vi "Create All Message Queues.vi"(8 "error in (no error)":errorcluster) -> (0 "error out":errorcluster, 3 "Message Queues out":T1)   [LabVIEW 2015, in "Message Queue.lvlib"]
doc: "This VI creates and initializes all the message queues for your application. If your application requires more than one message queue, right-click the \"Message Queues\" constant above and select Open Type Def. Add the new Message Queue(s) to the type definition, then initialize them in this VI."
uses:
  Message Queue.lvlib
  Message Cluster.ctl
  All Message Queues.ctl
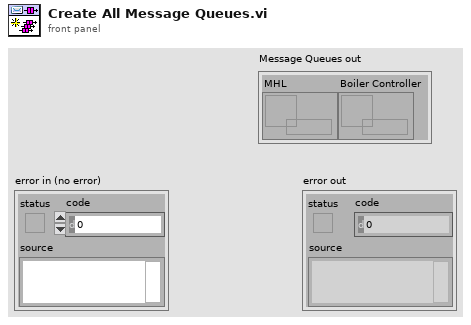
[diagram p1: front panel]
types:
  T1 = typedef "Message Queue.lvlib/All Message Queues.ctl" = cluster{"MHL":refnum<queue>, "Boiler Controller":refnum<queue>}
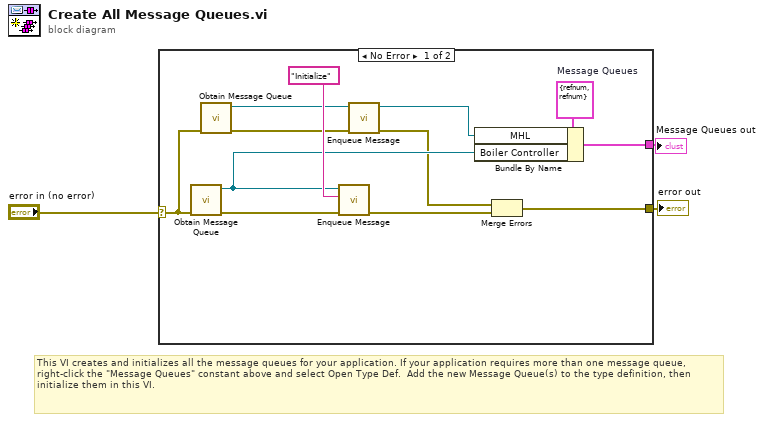
[diagram p0: block diagram]
diagram:
  # "This VI creates and initializes all the message queues for your application. If your application requires more than one message queue, right-click the \"Message Queues\" constant above and select Open Type Def.  Add the new Message Queue(s) to the type definition, then initialize them in this VI."
  n1 = case shown="No Error" "error in (no error)" {
    selector: "error in (no error)" -> [w6 w16]
    tunnel: [w9 w16] -> w3
    tunnel: [w11 _] -> w2
    frame No Error {
      w14 = T1 {"MHL"=refnum, "Boiler Controller"=refnum}  # Message Queues
      n2 = call "Obtain Message Queue.vi"("error in (no error)"=w6) -> ("error out"=w13:errorcluster, "Message Queue"=w10:refnum<queue>)  [unwired: 9 in]
      n3 = call "Obtain Message Queue.vi"("error in (no error)"=w6) -> ("error out"=w7:errorcluster, "Message Queue"=w5:refnum<queue>)  [unwired: 9 in]
      n4 = call "Enqueue Message.vi"("error in (no error)"=w13, "Message"="Initialize", "Message Queue"=w10) -> ("error out"=w15:errorcluster)  [unwired: 7 in, 1 out]
      n5 = call "Enqueue Message.vi"("error in (no error)"=w7, "Message Queue"=w5) -> ("error out"=w8:errorcluster, "dup Message Queue"=w4:refnum<queue>)  [unwired: 8 in]
      n6 = Bundle By Name(cluster=w14, "MHL"=w4, "Boiler Controller"=w10) -> (w11:T1)
      n7 = Merge Errors(w8, w15) -> (w9:errorcluster)
    }
    frame Error {
    }
  }
  "Message Queues out" <- w2
  "error out" <- w3
